vi "greenLocation.vi"() -> (0 "green_stop":bool, 1 "GREEN":T1, 2 "Green_Data":dbl[](array[numeric]))   [LabVIEW 2017]
panel:
  out "size":i32
  out "convex hull area":dbl
  out "Tayang":dbl
  out "Area":dbl
  out "Height":dbl
  out "Width":dbl
  out "Bottom":dbl
  out "Right":dbl
  out "Up":dbl
  out "Left":dbl
  out "CenterY":dbl
  out "CenterX":dbl
  out "Numeric":i32
  # "center x"
  # "center y"
  # "left"
  # "up"
  # "right"
  # "bot"
  # "width"
  # "height"
  # "tayang"
  # "area"
  # "convex hull area"
  # "img area"
  # "%area/img area"
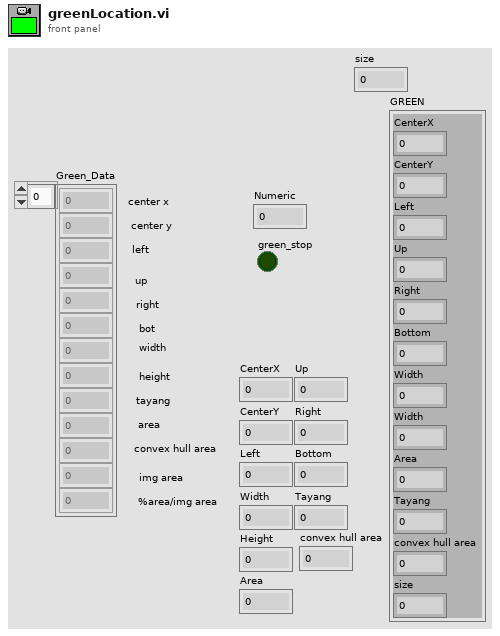
[diagram p1: front panel]
types:
  T1 = cluster{"CenterX":dbl, "CenterY":dbl, "Left":dbl, "Up":dbl, "Right":dbl, "Bottom":dbl, "Width":dbl, "Width":dbl, "Area":dbl, "Tayang":dbl, "convex hull area":dbl, "size":i32}
  T2 = typedef "IMAQ Image.ctl" = refnum<image>
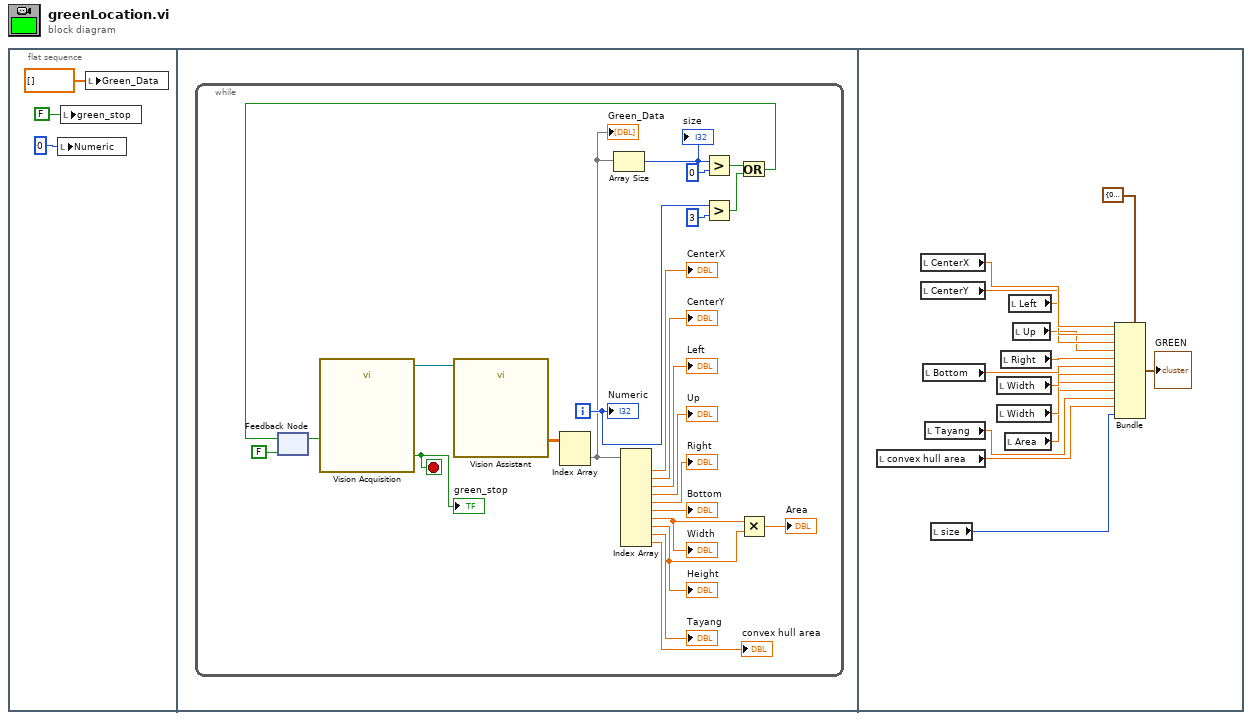
[diagram p0: block diagram]
diagram:
  n1 = flat-sequence {
    frame #0 {
      n2 = local write "Numeric"(0 ("Numeric")) -> ()
      n3 = local write "green_stop"(FALSE ("green_stop")) -> ()
      n4 = local write "Green_Data"(dbl[] [] ("Green_Data")) -> ()
    }
    frame #1 {
      n5 = while {
        i -> [w22]
        stop <- w16 stop-if-true
        n6 = feedback #1(FALSE) -> (w18:bool)
        n7 = call "Vision Acquisition"("Stop (F)"=w18) -> ("Image Out"=w27:T2, "Stopped"=w16:bool)  [unwired: 24 in, 1 out]
        "green_stop" <- w16
        n8 = call "Vision Assistant"("Image In"=w27) -> ("Particle Measurements (Pixels) (Particle Analysis 1)"=w26:dbl[][])  [unwired: 23 in, 3 out]
        n9 = Index Array(array=w26) -> (element=w4:dbl[])  [unwired: 2 in]
        "Green_Data" <- w4
        n10 = Array Size(array=w4) -> (size(s)=w25:i32)
        "size" <- w25
        n11 = Index Array(array=w4) -> (element #1=→"CenterX":dbl, element #2=→"CenterY":dbl, element #3=→"Left":dbl, element #4=→"Up":dbl, element #5=→"Right":dbl, element #6=→"Bottom":dbl, element #7=w15:dbl, element #8=w14:dbl, element #9=→"Tayang":dbl, element #10=→"convex hull area":dbl)  [unwired: 10 in]
        "Width" <- w15
        "Height" <- w14
        n12 = Greater?(x=w25, y=0) -> (0:w21:bool)
        n13 = Greater?(x=w22, y=3) -> (0:w20:bool)
        n14 = Or(x=w21, y=w20) -> (x .or. y?=w19:bool)
        n15 = feedback-in #1(w19) -> ()
        n16 = Multiply(x=w15, y=w14) -> (x*y=→"Area":dbl)
        "Numeric" <- w22
      }
    }
    frame #2 {
      n17 = local read "convex hull area"() -> (w31:dbl)
      n18 = local read "CenterX"() -> (w41:dbl)
      n19 = local read "CenterY"() -> (w40:dbl)
      n20 = local read "Bottom"() -> (w36:dbl)
      n21 = local read "Tayang"() -> (w32:dbl)
      n22 = local read "size"() -> (w30:i32)
      n23 = local read "Width"() -> (w35:dbl)
      n24 = local read "Width"() -> (w34:dbl)
      n25 = local read "Right"() -> (w37:dbl)
      n26 = local read "Area"() -> (w33:dbl)
      n27 = local read "Left"() -> (w39:dbl)
      n28 = local read "Up"() -> (w38:dbl)
      n29 = Bundle(cluster=T1 {"CenterX"=0.0, "CenterY"=0.0, "Left"=0.0, "Up"=0.0, "Right"=0.0, "Bottom"=0.0, "Width"=0.0, "Width"=0.0, "Area"=0.0, "Tayang"=0.0, "convex hull area"=0.0, "size"=0} ("output cluster"), "CenterX"=w41, "CenterY"=w40, "Left"=w39, "Up"=w38, "Right"=w37, "Bottom"=w36, "Width"=w35, "Width"=w34, "Area"=w33, "Tayang"=w32, "convex hull area"=w31, "size"=w30) -> (→"GREEN":T1)
    }
  }
